vi "Update Results.vi"(0 "measurement service v1 in":refnum<class "Measurement Service V1.lvclass">, 5 "measurement results":variant, 7 "measurement plugin service in":refnum<class "Measurement Plugin Service.lvclass">, 9 "gRPC ID in":T1, 11 "error in":errorcluster) -> (4 "measurement service v1 out":refnum<class "Measurement Service V1.lvclass">, 8 "measurement plugin service out":refnum<class "Measurement Plugin Service.lvclass">, 15 "error out":errorcluster)   [LabVIEW 2021, in "NI Measurement Plug-In SDK.lvlib" / "Measurement Service V1.lvclass"]
uses:
  Measurement Service V1.lvclass
  <vilib>/gRPC/LabVIEW gRPC Library/Shared/grpcId.ctl
  Measurement Plugin Service/Measurement Plugin Service.lvclass
  <vilib>/gRPC/LabVIEW gRPC Library/grpc-lvsupport-release.lvlib
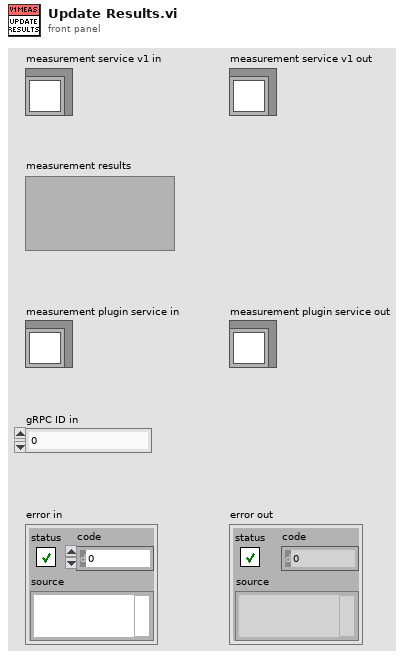
[diagram p1: front panel]
types:
  T1 = typedef "grpc-lvsupport-release.lvlib/grpcId.ctl" = u64
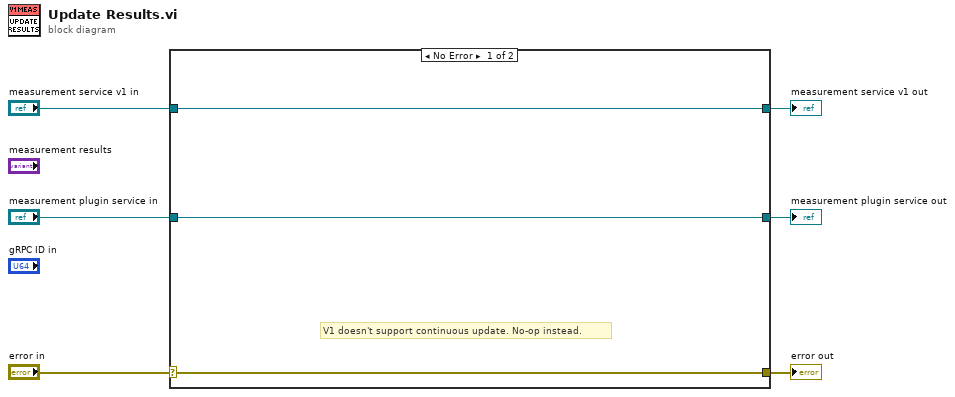
[diagram p0: block diagram]
diagram:
  n1 = case shown="No Error" "error in" {
    selector: "error in" -> [w7 w12]
    tunnel: [w7 w12] -> w5
    tunnel: [w9 w11] -> w3
    tunnel: "measurement service v1 in" -> [w9 w11]
    tunnel: "measurement plugin service in" -> [w8 w10]
    tunnel: [w8 w10] -> w1
    frame No Error {
      # "V1 doesn't support continuous update. No-op instead."
    }
    frame Error {
    }
  }
  "error out" <- w5
  "measurement service v1 out" <- w3
  "measurement plugin service out" <- w1
